vi "Wheel Power FGV.vi"(1 "New Power":dbl format="%#_13g", 2 "Swerve Number":enum16{"1", "2", "3", "4"}(ring), 3 "Action":enum16{"Set", "Get"}(ring)=enum."Get") -> (0 "Power":dbl)   [LabVIEW 2017, in "Huskie Swerve.lvlib"]
uses:
  Huskie Swerve.lvlib
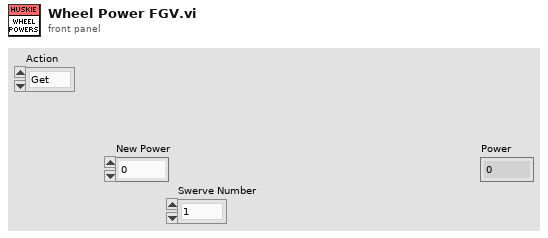
[diagram p1: front panel]
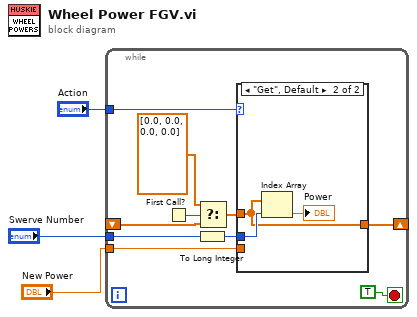
[diagram p0: block diagram]
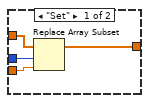
[diagram p2: hidden frame]
diagram:
  n1 = while {
    shift-right: [w8] -> _
    shift-left: _ -> [w4]
    tunnel: "New Power" -> [w9]
    tunnel: "Action" -> [w12]
    tunnel: "Swerve Number" -> [w11]
    stop <- TRUE stop-if-true
    n2 = First Call?() -> (First Call?: T/F=w7:bool)
    n3 = To Long Integer(number=w11) -> (32bit integer=w10:i32)
    n4 = Select(t=dbl[] [0.0, 0.0, 0.0, 0.0], s=w7, f=w4) -> (s? t:f=w5:dbl[])
    n5 = case shown="\"Get\", Default" w12 {
      tunnel: w5 -> [w17 w18]
      tunnel: w10 -> [w16 w20]
      tunnel: w9 -> [w15 _]
      tunnel: [w14 w18] -> w8
      frame "Set" {
        n6 = Replace Array Subset(array=w17, new element=w15, index=w16) -> (w14:dbl[])
      }
      frame "Get", Default {
        n7 = Index Array(array=w18, index=w20) -> (element=→"Power":dbl)
      }
    }
  }
